vi "Write timeout.vi"(10 "timeout":i32 min=0 max=5000, 11 "Network Endpoint in":refnum<class "Network Endpoint.lvclass">) -> (3 "Network Endpoint out":refnum<class "Network Endpoint.lvclass">)   [LabVIEW 2020, in "Network Endpoint.lvlib" / "Network Endpoint.lvclass"]
doc: "Sets the amount of time this actor will wait while attempting to create an endpoint (i.e. while waiting for a connection). If this value is too small, you may experience difficulty obtaining a connection. If it is too large, you may observe a delay when attempting to stop the actor. You must set this value prior to launching the actor.\n\nThis timeout limits both the time to wait for a connection and the time to wait for messages from the remote endpoint once a connection has been established."
uses:
  Network Endpoint.lvclass
  Network Endpoint.lvclass/Network Endpoint.ctl
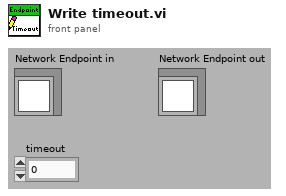
[diagram p1: front panel]
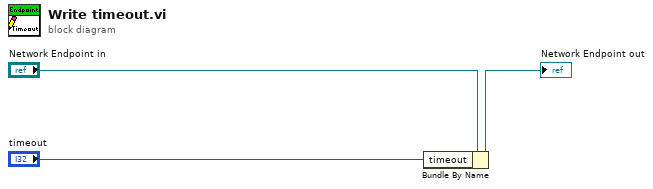
[diagram p0: block diagram]
diagram:
  n1 = Bundle By Name(cluster="Network Endpoint in", "timeout"="timeout") -> (→"Network Endpoint out":refnum<class "Network Endpoint.lvclass">)
